vi "Bypass Trigger Source.vi"(8 "error in (no error)":errorcluster, 11 "VISA resource name":refnum<visa-resource-name>) -> (0 "error out":errorcluster, 3 "VISA resource name out":refnum<visa-resource-name>)   [LabVIEW 2016, in "Keithley 2182.lvlib"]
doc: "Bypasses the control source when you do not wish to wait for the programmed event to occur. The instrument must be waiting at the control source for the event when this VI is used. Otherwise, an error occurs and the command is ignored.\n\n<b>Note:</b>\nWhen you set <b>Initiate Type</b> to <b>Continuous</b> in <b>Initiate VI</b>, and set <b>Trigger Source</b> to <b>Manual</b>, <b>Bus</b> or <b>External</b> in <b>Configure Trigger VI</b>, you can use this VI to bypass the control source."
uses:
  Keithley 2182.lvlib
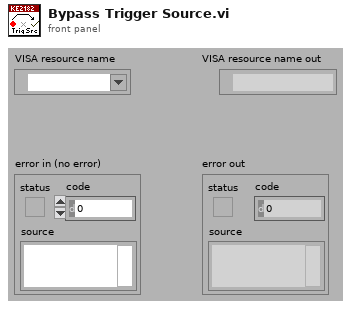
[diagram p1: front panel]
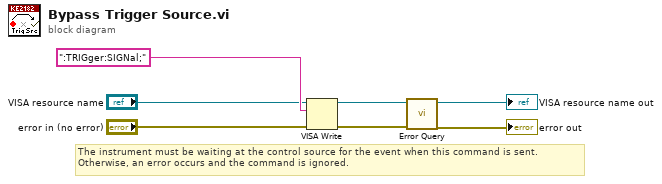
[diagram p0: block diagram]
diagram:
  # "The instrument must be waiting at the control source for the event when this command is sent. \nOtherwise, an error occurs and the command is ignored."
  n1 = VISA Write(VISA resource name="VISA resource name", write buffer=":TRIGger:SIGNal;", error in (no error)="error in (no error)") -> (VISA resource name out=w4:refnum<visa-resource-name>, error out=w3:errorcluster)  [unwired: 1 out]
  n2 = call "Error Query.vi"("error in (no error)"=w3, "VISA resource name"=w4) -> ("error out"=→"error out":errorcluster, "VISA resource name out"=→"VISA resource name out":refnum<visa-resource-name>)  [unwired: 6 in, 2 out]
